vi "手柄.vi"() -> ()   [LabVIEW 2017]
uses:
  <vilib>/Platform/TimedLoop/XDataNode/timing_clust.ctl
  <vilib>/Platform/TimedLoop/XDataNode/nitl_modes.ctl
  <vilib>/Platform/TimedLoop/XDataNode/wakeup.ctl
  <vilib>/Utility/inputDevices.llb/joystickAcquire.vi
  <vilib>/Utility/inputDevices.llb/closeJoystick.vi
  <vilib>/Platform/TimedLoop/XDataNode/XDataNode.xnode
  <vilib>/Platform/TimedLoop/XDataNode/XDNodeRunTimeDep.lvlib
panel:
  out "数组":dbl[](array[numeric])
  in  "最大值":dbl=32768.0
  in  "停止":bool
  out "direction info":T1 caption="方向信息"
  out "button info":T2 caption="按钮信息"
  out "axis info":T3 caption="坐标轴信息"
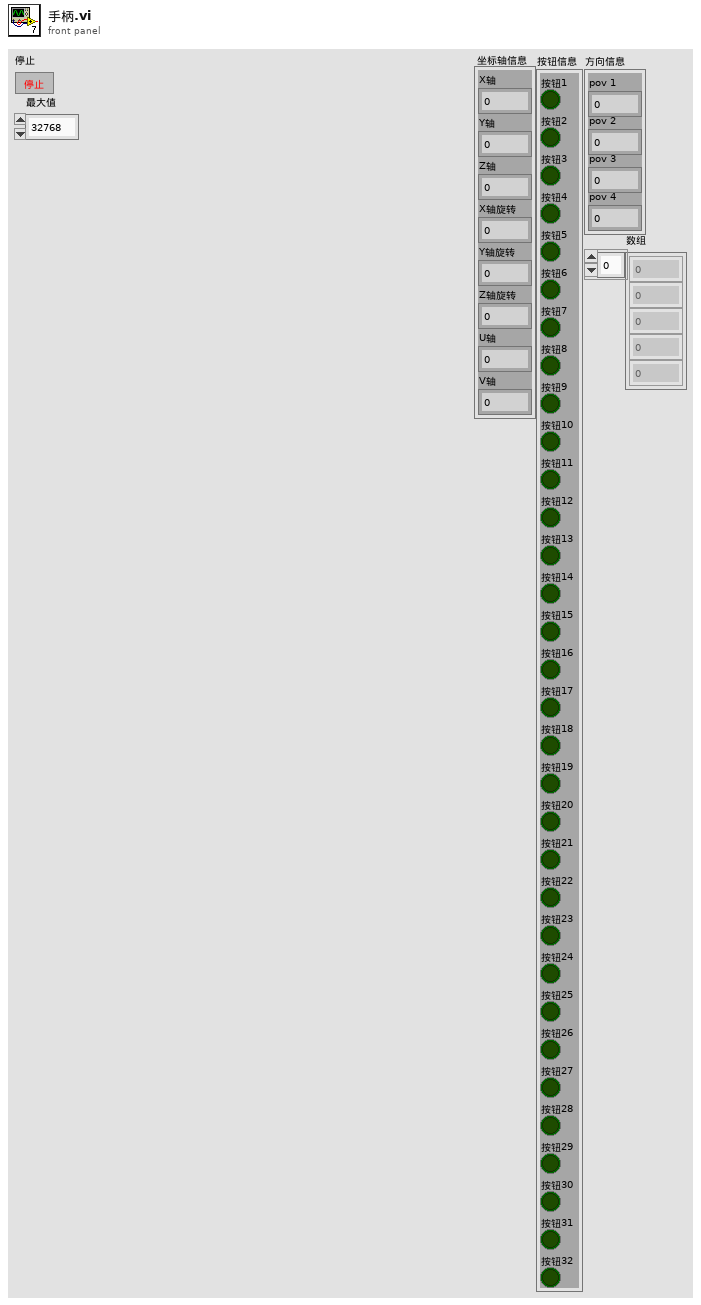
[diagram p1: front panel]
types:
  T1 = cluster{"pov 1":i32, "pov 2":i32, "pov 3":i32, "pov 4":i32}
  T2 = cluster{"button 1":bool, "button 2":bool, "button 3":bool, "button 4":bool, "button 5":bool, "button 6":bool, "button 7":bool, "button 8":bool, "button 9":bool, "button 10":bool, "button 11":bool, "button 12":bool, "button 13":bool, "button 14":bool, "button 15":bool, "button 16":bool, "button 17":bool, "button 18":bool, "button 19":bool, "button 20":bool, "button 21":bool, "button 22":bool, "button 23":bool, "button 24":bool, "button 25":bool, "button 26":bool, "button 27":bool, "button 28":bool, "button 29":bool, "button 30":bool, "button 31":bool, "button 32":bool}
  T3 = cluster{"X axis":i32, "Y axis":i32, "Z axis":i32, "X axis rotation":i32, "Y axis rotation":i32, "Z axis rotation":i32, "U axis":i32, "V axis":i32}
  T4 = cluster{"axes total":u32, "buttons total":u32, "pov total":u32, "device name":string}[]
  T5 = typedef "XDNodeRunTimeDep.lvlib/timing_clust.ctl" = cluster{"Expected End [f-1]":u64, "Actual End [f-1]":u64, "Finished Late? [f-1]":bool, "Expected End [i-1]":u64, "Actual End [i-1]":u64, "Finished Late? [i-1]":bool, "Expected Start [i]":u64, "Actual Start [i]":u64, "Expected Start [f]":u64, "Actual Start [f]":u64, "Source Name":string, "Structure Name":string, "Period":i64, "Deadline":i64, "Offset":i64, "Start":i64, "Priority":i32, "Timeout":i32, "Mode":T6, "Wakeup Reason":T7, "Error":errorcluster, "Source Type":string, "Secondary Source Type":string, "Global End Time":u64, "Global Start Time":u64, "Frame Duration":u64, "Iteration Duration":u64, "Assigned CPU":i32, "I/O Scan Engine Mode":u32}
  T6 = typedef "XDNodeRunTimeDep.lvlib/nitl_modes.ctl" = enum32{"No Change", "Process missed periods, maintain original phase", "Discard missed periods, maintain original phase", "Process missed periods, ignore original phase", "Discard missed periods, ignore original phase"}
  T7 = typedef "XDNodeRunTimeDep.lvlib/wakeup.ctl" = enum32{"Normal", "Aborted", "Asynchronous wakeup", "Timing source error", "Timed loop error", "Timeout"}
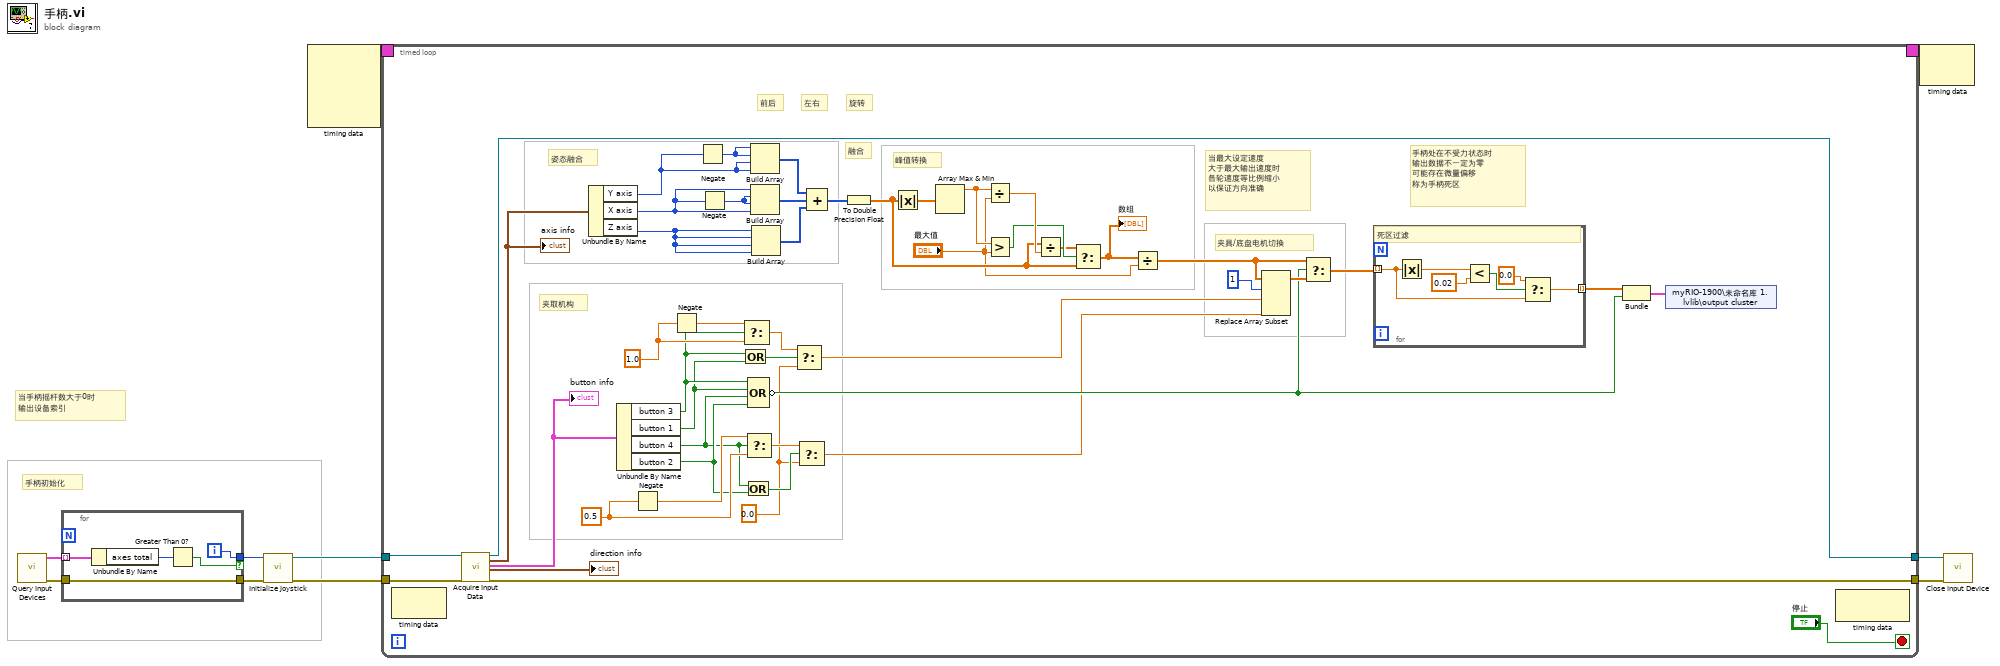
[diagram p0: block diagram]
diagram:
  # "当手柄摇杆数大于0时\n输出设备索引"
  # "手柄初始化"
  n1 = call <vilib>:"Query Input Devices.vi"() -> ("error out"=w3:errorcluster, "joystick info"=w8:T4)  [unwired: 8 in, 2 out]
  n2 = for {
    tunnel: w8 -> [w14] mode=indexing
    tunnel: [w13] -> w7 if=w12
    tunnel: w3 -> [w11]
    tunnel: [w11] -> w2
    i -> [w13]
    n3 = Unbundle By Name(w14) -> ("axes total"=w15:u32)
    n4 = Greater Than 0?(x=w15) -> (x > 0?=w12:bool)
  }
  n5 = call <vilib>:"Initialize Joystick.vi"("error in (no error)"=w2, "device index"=w7) -> ("error out"=w4:errorcluster, "device ID"=w6:refnum<k1>)  [unwired: 8 in]
  n6 = node-c288() -> (w10:T5)  [unwired: 4 in]
  n7 = timed-loop {
    timing: w10 -> [_]
    timing-out: [_] -> w9
    tunnel: w6 -> [w62]
    tunnel: [w61] -> w5
    tunnel: w4 -> [w60]
    tunnel: [w59] -> w1
    stop <- "停止" stop-if-true
    w22 = 0.0
    w35 = 0.5
    w36 = 1.0
    # "融合"
    # "旋转"
    # "左右"
    # "前后"
    # "手柄处在不受力状态时\n输出数据不一定为零\n可能存在微量偏移\n称为手柄死区"
    # "当最大设定速度\n大于最大输出速度时\n各轮速度等比例缩小\n以保证方向准确"
    # "夹具/底盘电机切换"
    # "夹取机构"
    # "峰值转换"
    # "姿态融合"
    n8 = node-c288() -> ()  [unwired: 1 in, 1 out]
    n9 = call-poly <vilib>:"Acquire Input Data.vi"("device ID"=w62, "error in (no error)"=w60) -> ("device ID"=w61:refnum<k1>, "axis info"=w56:T3, "button info"=w55:T2, "direction info"=→"direction info":T1, "error out"=w59:errorcluster)  [unwired: 13 in]
    "axis info" <- w56
    "button info" <- w55
    n10 = Unbundle By Name(w56) -> ("Y axis"=w54:i32, "X axis"=w40:i32, "Z axis"=w53:i32)
    n11 = Unbundle By Name(w55) -> ("button 3"=w30:bool, "button 1"=w29:bool, "button 4"=w25:bool, "button 2"=w26:bool)
    n12 = Negate(x=w35) -> (-x=w34:dbl)
    n13 = Negate(x=w36) -> (-x=w37:dbl)
    n14 = Negate(x=w54) -> (-x=w42:i32)
    n15 = Negate(x=w40) -> (-x=w41:i32)
    n16 = Or(x=w30, y=w29) -> (x .or. y?=w28:bool)
    n17 = Select(t=w37, s=w30, f=w36) -> (s? t:f=w27:dbl)
    n18 = Or(x=w25, y=w26) -> (x .or. y?=w24:bool)
    n19 = Select(t=w34, s=w25, f=w35) -> (s? t:f=w23:dbl)
    n20 = Compound Arithmetic op=OR ("复合运算")(w30, w29, w25, w26) -> (invert w31:bool)
    n21 = Build Array(w42, w42, w54, w54) -> (w52:i32[])
    n22 = Build Array(w40, w41, w41, w40) -> (w51:i32[])
    n23 = Build Array(w53, w53, w53, w53) -> (w43:i32[])
    n24 = Select(t=w27, s=w28, f=w22) -> (s? t:f=w21:dbl)
    n25 = Select(t=w23, s=w24, f=w22) -> (s? t:f=w20:dbl)
    n26 = Compound Arithmetic op=ADD(w52, w51, w43) -> (w49:i32[])
    n27 = To Double Precision Float(number=w49) -> (double precision float=w45:dbl[])
    n28 = Absolute Value(x=w45) -> (abs(x)=w44:dbl[])
    n29 = Array Max & Min(array=w44) -> (max value=w48:dbl)  [unwired: 3 out]
    n30 = Divide(x=w48, y="最大值") -> (x/y=w50:dbl)
    n31 = Greater?(x=w48, y="最大值") -> (0:w47:bool)
    n32 = Divide(x=w45, y=w50) -> (x/y=w46:dbl[])
    n33 = Select(t=w46, s=w47, f=w45) -> (s? t:f=w38:dbl[])
    "数组" <- w38
    n34 = Divide(x=w38, y="最大值") -> (x/y=w33:dbl[])
    n35 = Replace Array Subset(array=w33, new element #1=w21, index #1=1 ("索引"), new element #2=w20) -> (w32:dbl[])  [unwired: 1 in]
    n36 = Select(t=w33, s=w31, f=w32) -> (s? t:f=w17:dbl[])
    n37 = for {
      tunnel: w17 -> [w65] mode=indexing
      tunnel: [w63] -> w16 mode=indexing
      # "死区过滤"
      n38 = Absolute Value(x=w65) -> (abs(x)=w68:dbl)
      n39 = Less?(x=w68, y=0.02) -> (x < y?=w66:bool)
      n40 = Select(t=0.0, s=w66, f=w65) -> (s? t:f=w63:dbl)
    }
    n41 = Bundle(w16, w31) -> (w18:cluster{dbl[], bool})  [unwired: 1 in]
    n42 = shared-variable "myRIO-1900\\未命名库 1.lvlib\\output cluster"(w18) -> ()  [unwired: 1 in, 1 out]
    n43 = node-c288() -> ()  [unwired: 1 in, 1 out]
  }
  n44 = node-c288(w9) -> ()  [unwired: 1 out]
  n45 = call-poly <vilib>:"Close Input Device.vi"("error in (no error)"=w1, "device ID"=w5) -> ()  [unwired: 8 in, 1 out]
